vi "Close Project References.vi"(8 "error in (no error)":errorcluster, 10 "Save All":bool=TRUE, 11 "LabVIEW Build Script in":refnum<class "LabVIEW Build Script.lvclass">) -> (0 "error out":errorcluster, 3 "LabVIEW Build Script out":refnum<class "LabVIEW Build Script.lvclass">)   [LabVIEW 2021, in "LabVIEW Build Script.lvclass"]
uses:
  LabVIEW Build Script.lvclass
  LabVIEW Build Script.lvclass/LabVIEW Build Script.ctl
  <vilib>/CIF Foundation/CIF LabVIEW Scripting/LV Scripting/LV Scripting Utilities.lvlib
  <vilib>/CIF Foundation/CIF LabVIEW Scripting/LV Scripting/Typedef/Target References.ctl
  <vilib>/CIF Foundation/CIF LabVIEW Scripting/LV Scripting/Typedef/Library Map.ctl
  <vilib>/CIF Foundation/CIF LabVIEW Scripting/LV Scripting/Typedef/VI Map.ctl
  <vilib>/CIF Foundation/CIF LabVIEW Scripting/LV Scripting/Typedef/BuildSpec Map.ctl
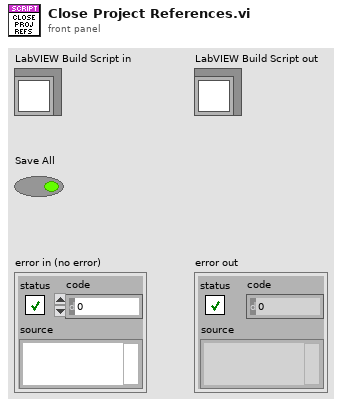
[diagram p1: front panel]
types:
  T1 = typedef "LV Scripting Utilities.lvlib/BuildSpec Map.ctl" = map{string, refnum<vi>}
  T2 = typedef "LV Scripting Utilities.lvlib/VI Map.ctl" = map{string, refnum<vi>}
  T3 = typedef "LV Scripting Utilities.lvlib/Library Map.ctl" = map{string, refnum<vi>}
  T4 = typedef "LV Scripting Utilities.lvlib/Target References.ctl" = cluster{"Target Reference":refnum<vi>, "VI References":refnum<vi>[], "Library References":refnum<vi>[], "Build References":refnum<vi>[]}
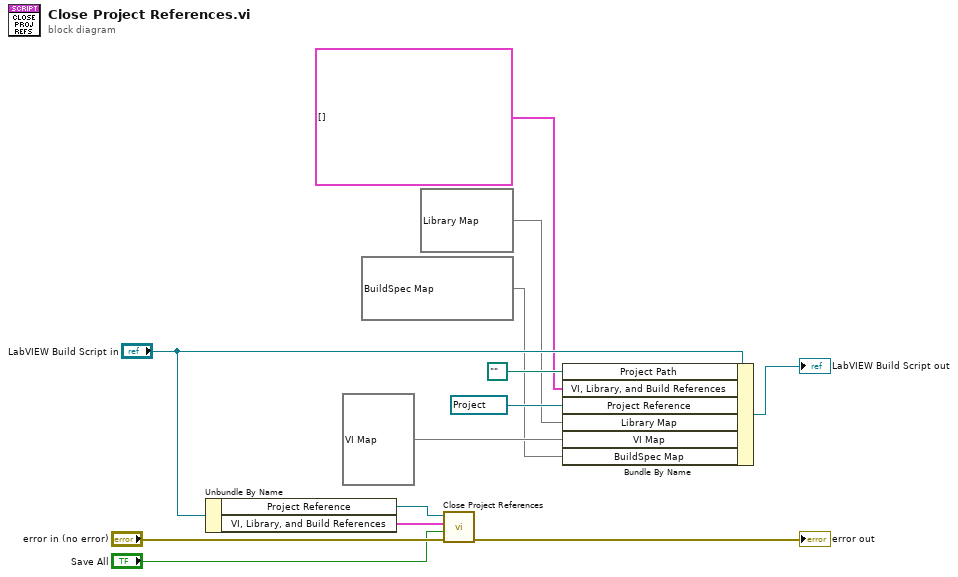
[diagram p0: block diagram]
diagram:
  n1 = Unbundle By Name("LabVIEW Build Script in") -> ("Project Reference"=w11:refnum<vi>, "VI, Library, and Build References"=w10:T4[])
  n2 = call <vilib>:"Close Project References.vi"("error in"="error in (no error)", "Save All"="Save All", "VI, Library, and Build References"=w10, "Project Reference"=w11) -> ("error out"=→"error out":errorcluster)  [unwired: 7 in]
  n3 = Bundle By Name(cluster="LabVIEW Build Script in", "Project Path"=path "", "VI, Library, and Build References"=T4[] [], "Project Reference"=refnum<vi> refnum, "Library Map"=T3 {}, "VI Map"=T2 {}, "BuildSpec Map"=T1 {}) -> (→"LabVIEW Build Script out":refnum<class "LabVIEW Build Script.lvclass">)
